vi "ConvertImperialLength_viaEventStructure.vi"() -> ()   [LabVIEW 2024]
panel:
  in  "stop":bool
  out "Numeric 2":dbl
  in  "Mile Button 4":bool
  in  "Yard  Button 3":bool
  in  "Feet Button 2":bool
  in  "Inch Button":bool
  in  "Numeric":dbl
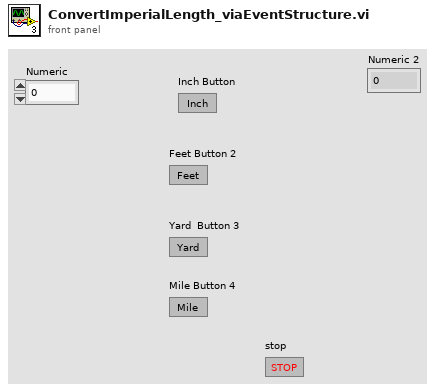
[diagram p1: front panel]
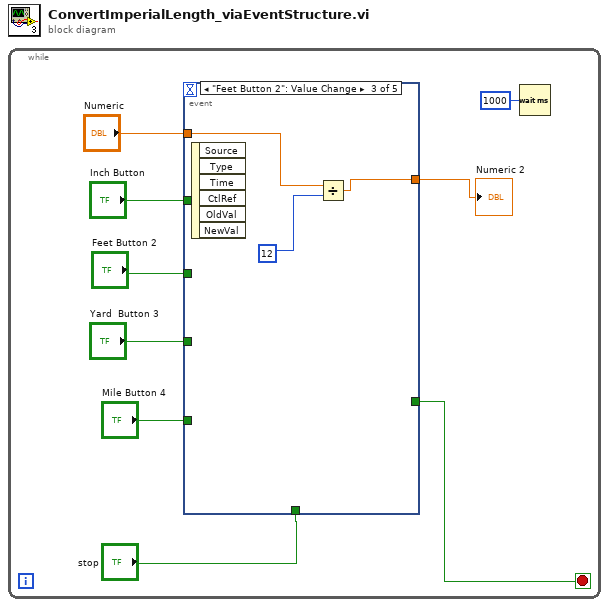
[diagram p0: block diagram]
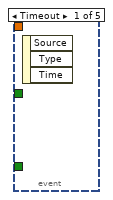
[diagram p2: hidden frame]
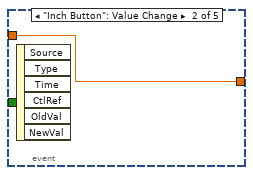
[diagram p3: hidden frame]
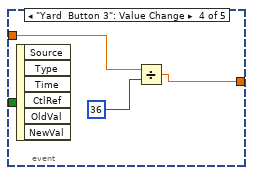
[diagram p4: hidden frame]
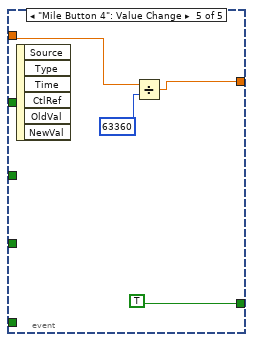
[diagram p5: hidden frame]
diagram:
  n1 = while {
    stop <- w1 stop-if-true
    n2 = event shown="[2] \"Feet Button 2\": Value Change" {
      selector: _ -> [_ _ _ _ _]
      dyn-events: _ -> [_ _ _ _ _]
      timeout: _ -> [_ _ _ _ _]
      tunnel: "Numeric" -> [_ w11 w14 w17 w21]
      tunnel: "Inch Button" -> [_ _ _ _ _]
      tunnel: [w10 _ _ _ _] -> _
      tunnel: "Feet Button 2" -> [w10 _ _ _ _]
      tunnel: "Yard  Button 3" -> [_ _ _ _ _]
      tunnel: "Mile Button 4" -> [_ _ _ _ _]
      tunnel: [_ w11 w12 w15 w20] -> w4
      tunnel: "stop" -> [_ _ _ _ _]
      tunnel: [_ _ _ _ TRUE] -> w1
      event Timeout {
        n3 = event-data() -> ()  [unwired: 1 in, 3 out]
      }
      event "Inch Button": Value Change {
        n4 = event-data() -> ()  [unwired: 1 in, 6 out]
      }
      event "Feet Button 2": Value Change {
        n5 = event-data() -> ()  [unwired: 1 in, 6 out]
        n6 = Divide(x=w14, y=12) -> (x/y=w12:dbl)
      }
      event "Yard  Button 3": Value Change {
        n7 = event-data() -> ()  [unwired: 1 in, 6 out]
        n8 = Divide(x=w17, y=36) -> (x/y=w15:dbl)
      }
      event "Mile Button 4": Value Change {
        n9 = event-data() -> ()  [unwired: 1 in, 6 out]
        n10 = Divide(x=w21, y=63360) -> (x/y=w20:dbl)
      }
    }
    "Numeric 2" <- w4
    n11 = Wait (ms)(milliseconds to wait=u32 1000) -> ()  [unwired: 1 out]
  }
